vi "z-stack acquistion.vi"() -> ()   [LabVIEW 2014]
uses:
  SubVIs/Initilize Globals.vi
  Stage Control/Stage SubVis/move stage.ctl
  SubVIs/ctt's/image acquisition 3.ctl
  SubVIs/ctt's/image acquisiton 4.ctl
panel:
  in  "stage settle time (ms)":u32
  in  "stack half-width":u32
  in  "focus step (um)":dbl
  in  "Acquisition Protocol":T1(array[cluster])
  in  "Max. number of acquisition files":i8(slide)=10 scale=0.0..50.0
  in  "Cycle Interval (s)":dbl format="%_3f"
  in  "Image Size":T2={"H Bin"=1.0, "V Bin"=1.0, "Left"=1.0, "Right"=1024.0, "Top"=1.0, "Bottom"=1024.0} {"V Bin" min=0.0; "H Bin" min=0.0 step=1.0}
  in  "Acquisition Parameters":T3={"Readout Mode"=enum."Image", "Set Acquisition Mode"=enum."Single Scan", "Trigger Mode"=enum."Internal", "Exposure Time (s)"=1.0, "Accumulation Cycle (s)"=1.0, "Kinetic Cycle Time (s)"=1.0, "Number of Kinetics"=1, "Number of Accumulations"=1, "Set VS Speed"=1, "Pixel Rate"=enum."Standard CCD 3 Mhz 14 bits", "V Shift Amplitude"=enum."+1", "Preamp Gain"=enum."1.0"}
  # "Z-stack parameters"
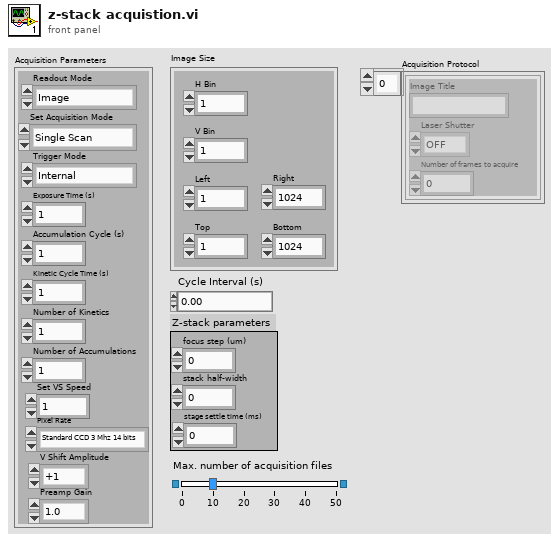
[diagram p1: front panel]
types:
  T1 = cluster{"Image Title":string, "Laser Shutter":enum32{"GFP", "Cy3 Long Pass", "Cy3", "Cy5", "OFF"}, "Number of frames to acquire":i32}[]
  T2 = typedef "image acquisiton 4.ctl" = cluster{"H Bin":dbl, "V Bin":dbl, "Left":dbl, "Right":dbl, "Top":dbl, "Bottom":dbl}
  T3 = typedef "image acquisition 3.ctl" = cluster{"Readout Mode":enum16{"Full Vertical Binning", "Multi-Track", "Random-Track", "Single-Track", "Image"}, "Set Acquisition Mode":enum16{"(do nothing)", "Single Scan", "Accumulate", "Kinetics", "Fast Kinetics", "Run till abort"}, "Trigger Mode":enum16{"Internal", "External"}, "Exposure Time (s)":dbl, "Accumulation Cycle (s)":dbl, "Kinetic Cycle Time (s)":dbl, "Number of Kinetics":i32, "Number of Accumulations":i32, "Set VS Speed":i32, "Pixel Rate":enum16{"EM CCD 10 Mhz 14 bits", "EM CCD 5 Mhz 14 bits", "EM CCD 3 Mhz 14 bits", "EM CCD 1 Mhz 16 bits", "Standard CCD 3 Mhz 14 bits", "Standard CCD 1 Mhz 16 bits"}, "V Shift Amplitude":enum16{"normal", "+1", "+2", "+3", "+4"}, "Preamp Gain":enum16{"1.0", "2.4", "5.0"}}
  T4 = cluster{"Frame Size (bytes)":i32, "Max Time (min)":i32, "Max Frames":i32, "Frames per acquisition file":i32, "Max time (s)":i32, "Max Space Req'd. (Gb)":dbl}
  T5 = typedef "acquisition control.ctl" = cluster{"H Bin":dbl, "V Bin":dbl, "Left":dbl, "Right":dbl, "Top":dbl, "Bottom":dbl}
  T6 = typedef "move stage.ctl" = cluster{"dx (um) (0 -> ignore)":ext, "dy (um) (0 -> ignore)":ext, "dz (um) (0 -> ignore)":ext, "Re-center x,y":bool, "Re-center z":bool, "x (um) (-1 -> ignore)":dbl, "y (um) (-1 -> ignore)":dbl, "z (um) (-1 -> ignore)":dbl}
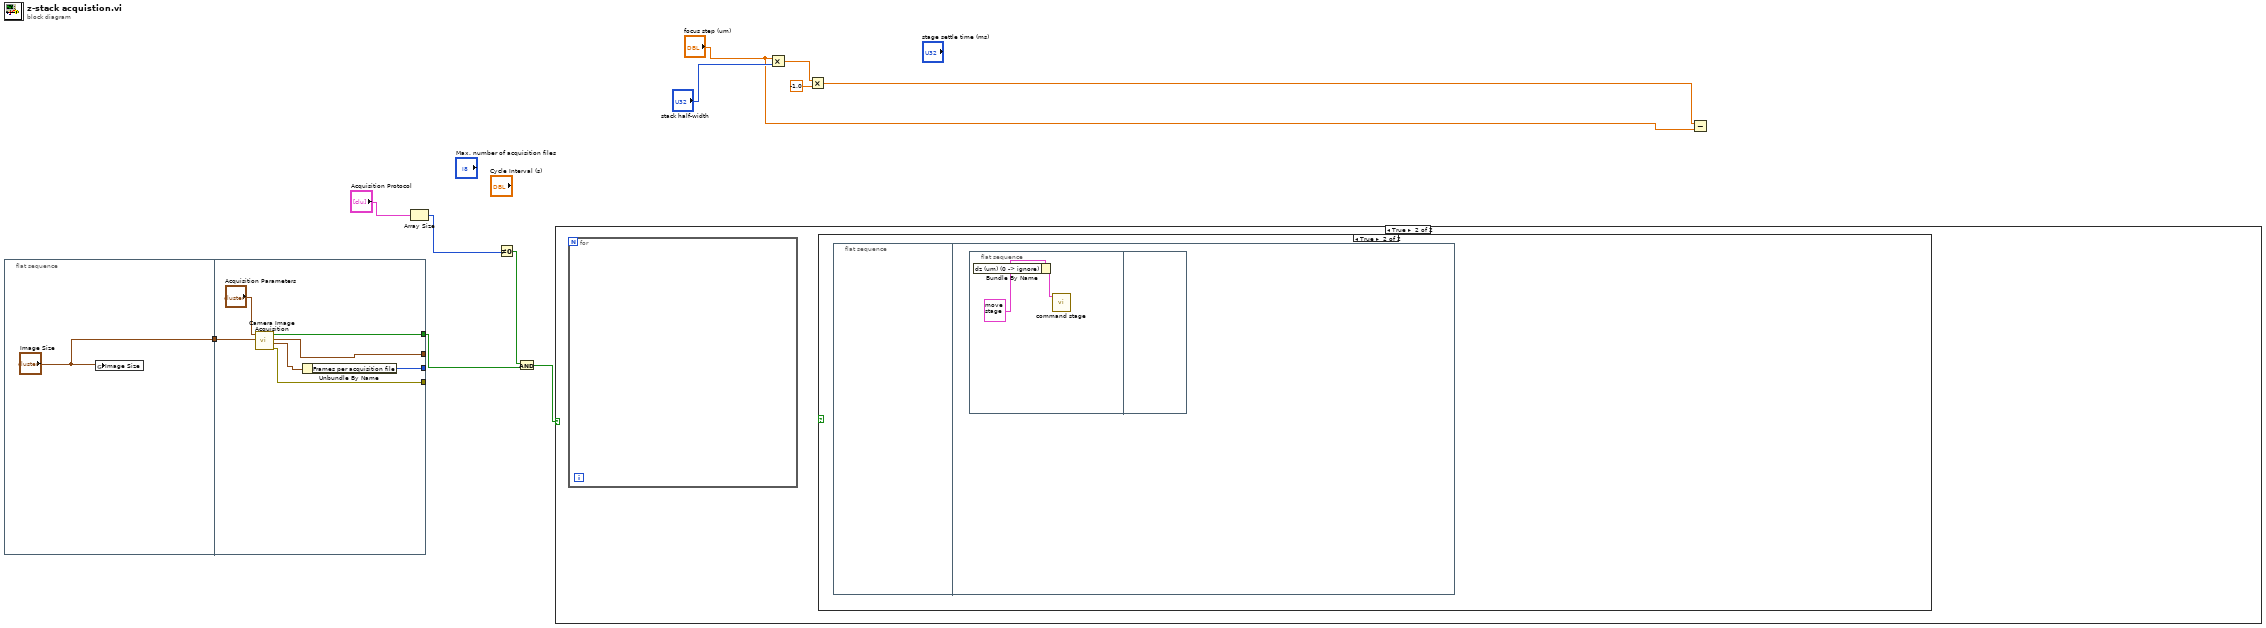
[diagram p0: block diagram]
diagram:
  n1 = flat-sequence {
    tunnel: ["Image Size"] -> w11
    tunnel: w11 -> [w19]
    tunnel: [w17] -> w7
    tunnel: [w16] -> _
    tunnel: [w15] -> _
    tunnel: [w13] -> _
    frame #0 {
      n2 = global write "Initilize Globals.vi" "Image Size"("Image Size") -> ()
    }
    frame #1 {
      n3 = call "Camera Image Acquisition.vi"("Image Size"=w19, "Acquisition Parameters"="Acquisition Parameters") -> ("Error Out"=w16:errorcluster, "File properties"=w14:T4, "Image Size 2"=w15:T5, "Continue with acq?"=w17:bool)  [unwired: 6 in]
      n4 = Unbundle By Name(w14) -> ("Frames per acquisition file"=w13:i32)
    }
  }
  n5 = Array Size(array="Acquisition Protocol") -> (size(s)=w9:i32)
  n6 = Not Equal To 0?(x=w9) -> (x != 0?=w8:bool)
  n7 = And(x=w8, y=w7) -> (x .and. y?=w6:bool)
  n8 = case shown="True" w6 {
    frame False {
    }
    frame True {
      n9 = for {
      }
      n10 = case shown="True" {
        selector: _ -> [_ _]
        frame False {
        }
        frame True {
          n11 = flat-sequence {
            frame #0 {
            }
            frame #1 {
              n12 = flat-sequence {
                frame #0 {
                  n13 = Bundle By Name(cluster=T6 {"dx (um) (0 -> ignore)"=0.0, "dy (um) (0 -> ignore)"=0.0, "dz (um) (0 -> ignore)"=0.0, "Re-center x,y"=FALSE, "Re-center z"=FALSE, "x (um) (-1 -> ignore)"=-1.0, "y (um) (-1 -> ignore)"=-1.0, "z (um) (-1 -> ignore)"=-1.0} ("Command Stage")) -> (w20:T6)  [unwired: 1 in]
                  n14 = call "command stage.vi"("Command Stage"=w20) -> ()  [unwired: 10 in, 1 out]
                }
                frame #1 {
                }
              }
            }
          }
        }
      }
    }
  }
  n15 = Multiply(x="focus step (um)", y="stack half-width") -> (x*y=w4:dbl)
  n16 = Multiply(x=w4, y=-1.0) -> (x*y=w1:dbl)
  n17 = Subtract(x=w1, y="focus step (um)") -> ()  [unwired: 1 out]
